vi "Dual-move-motor.vi"() -> ()   [LabVIEW 2014]
panel:
  in  "stop 2":bool
  out "pfPosition 2":sgl
  out "Numeric 2":i32
  out "Motor Y\nLigado 2":bool=TRUE
  out "Numeric":i32
  out "pfPosition":sgl
  in  "stop":bool
  out "Motor Y\nLigado":bool=TRUE
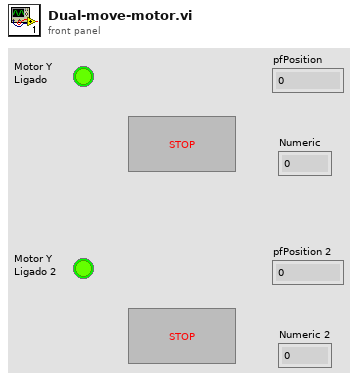
[diagram p1: front panel]
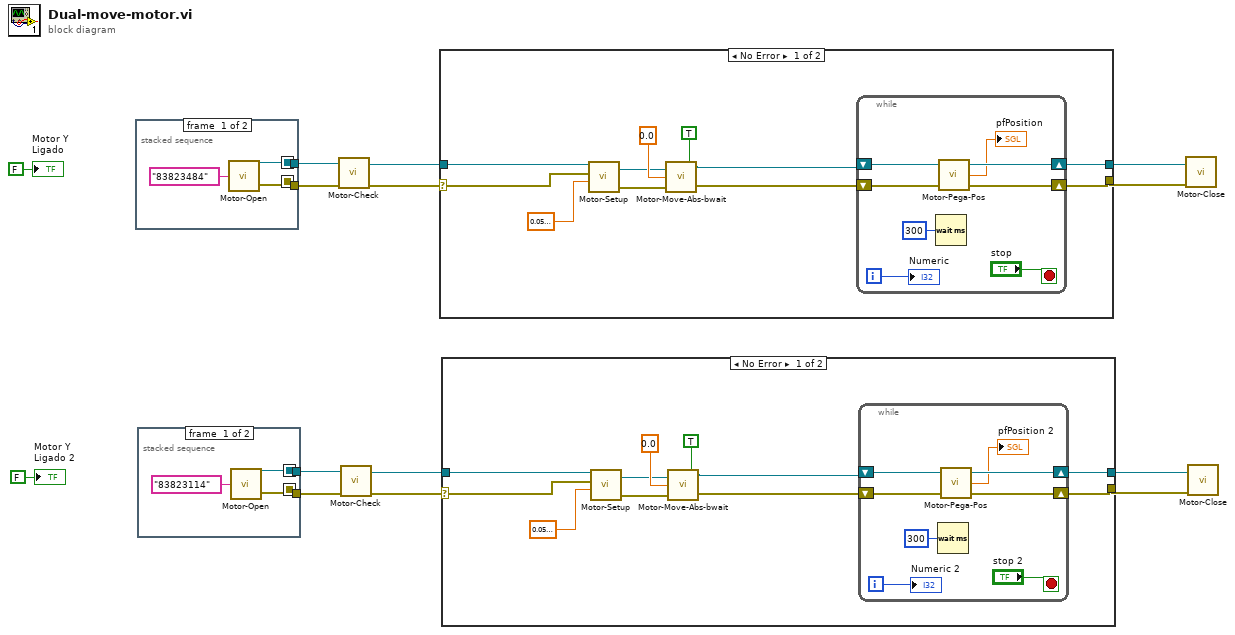
[diagram p0: block diagram]
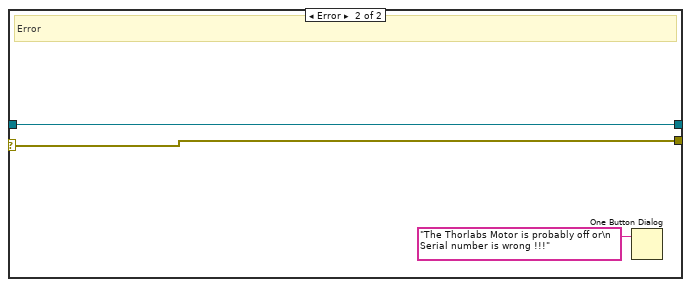
[diagram p2: hidden frame]
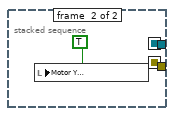
[diagram p3: hidden frame]
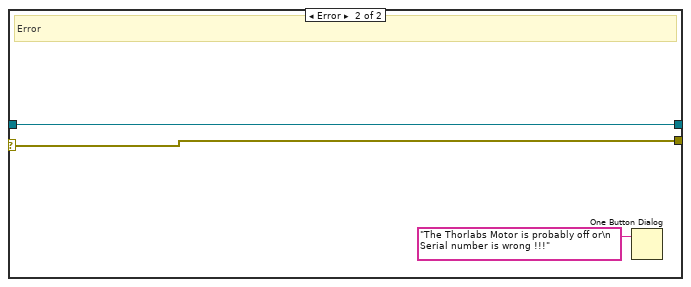
[diagram p4: hidden frame]
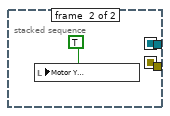
[diagram p5: hidden frame]
diagram:
  n1 = stacked-sequence {
    seq-local: [w17 _] -> [_ w20]
    seq-local: [w16 _] -> [_ w19]
    tunnel: [_ w20] -> w11
    tunnel: [_ w19] -> w10
    frame #0 {
      n2 = call "Motor-Open.vi"("S/N Motor"="83823484") -> ("MG17Motor 2"=w17:refnum<k7>, "error out"=w16:errorcluster)
    }
    frame #1 {
      n3 = local write "Motor Y\nLigado"(TRUE ("Motor3\nLigado")) -> ()
    }
  }
  n4 = stacked-sequence {
    seq-local: [w23 _] -> [_ w26]
    seq-local: [w22 _] -> [_ w25]
    tunnel: [_ w26] -> w4
    tunnel: [_ w25] -> w3
    frame #0 {
      n5 = call "Motor-Open.vi"("S/N Motor"="83823114") -> ("MG17Motor 2"=w23:refnum<k7>, "error out"=w22:errorcluster)
    }
    frame #1 {
      n6 = local write "Motor Y\nLigado 2"(TRUE ("Motor3\nLigado")) -> ()
    }
  }
  n7 = call "Motor-Check.vi"("error in (no error)"=w10, "Automation Refnum in"=w11) -> ("error out"=w8:errorcluster, "Automation Refnum out"=w9:refnum<k7>)  [unwired: 8 in]
  n8 = call "Motor-Check.vi"("error in (no error)"=w3, "Automation Refnum in"=w4) -> ("error out"=w1:errorcluster, "Automation Refnum out"=w2:refnum<k7>)  [unwired: 8 in]
  n9 = case shown="No Error" w8 {
    selector: w8 -> [w29 w46]
    tunnel: w9 -> [w28 w47]
    tunnel: [w37 w47] -> w13
    tunnel: [w36 w46] -> w12
    frame No Error {
      n10 = call "Motor-Setup.vi"("Velocidade"=sgl 0.05, "error"=w29, "MG17Motor A"=w28) -> ("error out"=w31:errorcluster, "MG17Motor out"=w30:refnum<k7>)  [unwired: 1 in]
      n11 = call "Motor-Move-Abs-bwait.vi"("bWait"=TRUE, "error"=w31, "Posição"=sgl 0.0, "MG17Motor A"=w30) -> ("error out"=w35:errorcluster, "MG17Motor out"=w34:refnum<k7>)
      n12 = while {
        shift-right: [w43] -> w37
        shift-left: w34 -> [w45]
        shift-right: [w42] -> w36
        shift-left: w35 -> [w44]
        i -> [w38]
        stop <- "stop" stop-if-true
        n13 = Wait (ms)(milliseconds to wait=u32 300) -> ()  [unwired: 1 out]
        n14 = call "Motor-Pega-Pos.vi"("MG17Motor 2"=w45, "error out"=w44) -> ("MG17Motor 3"=w43:refnum<k7>, "pfPosition"=→"pfPosition":sgl, "error out 2"=w42:errorcluster)
        "Numeric" <- w38
      }
    }
    frame Error {
      # "Error"
      n15 = One Button Dialog(message="The Thorlabs Motor is probably off or\n Serial number is wrong !!!") -> ()  [unwired: 1 in, 1 out]
    }
  }
  n16 = case shown="No Error" w1 {
    selector: w1 -> [w51 w68]
    tunnel: w2 -> [w50 w69]
    tunnel: [w59 w69] -> w6
    tunnel: [w58 w68] -> w5
    frame No Error {
      n17 = call "Motor-Setup.vi"("Velocidade"=sgl 0.05, "error"=w51, "MG17Motor A"=w50) -> ("error out"=w53:errorcluster, "MG17Motor out"=w52:refnum<k7>)  [unwired: 1 in]
      n18 = call "Motor-Move-Abs-bwait.vi"("bWait"=TRUE, "error"=w53, "Posição"=sgl 0.0, "MG17Motor A"=w52) -> ("error out"=w57:errorcluster, "MG17Motor out"=w56:refnum<k7>)
      n19 = while {
        shift-right: [w65] -> w59
        shift-left: w56 -> [w67]
        shift-right: [w64] -> w58
        shift-left: w57 -> [w66]
        i -> [w60]
        stop <- "stop 2" stop-if-true
        n20 = Wait (ms)(milliseconds to wait=u32 300) -> ()  [unwired: 1 out]
        n21 = call "Motor-Pega-Pos.vi"("MG17Motor 2"=w67, "error out"=w66) -> ("MG17Motor 3"=w65:refnum<k7>, "pfPosition"=→"pfPosition 2":sgl, "error out 2"=w64:errorcluster)
        "Numeric 2" <- w60
      }
    }
    frame Error {
      # "Error"
      n22 = One Button Dialog(message="The Thorlabs Motor is probably off or\n Serial number is wrong !!!") -> ()  [unwired: 1 in, 1 out]
    }
  }
  n23 = call "Motor-Close.vi"("error out"=w12, "MG17Motor 3"=w13) -> ()  [unwired: 1 in]
  n24 = call "Motor-Close.vi"("error out"=w5, "MG17Motor 3"=w6) -> ()  [unwired: 1 in]
  "Motor Y\nLigado" <- FALSE ("Motor Y\nLigado")
  "Motor Y\nLigado 2" <- FALSE ("Motor Y\nLigado")
